vi "go to abort.vi"(0 "system status in":T2={"system state"=enum."Empty & Closed", "fuel level"=0.0, "LOX level"=0.0, "system warnings"={"oxidizer overpress"=FALSE, "oxidizer leak"=FALSE, "fuel overpress"=FALSE, "fuel leak"=FALSE}, "valves"={"fuel load"=FALSE, "fuel return"=FALSE, "fuel comb"=FALSE, "fuel dump"=FALSE, "LOX load"=FALSE, "LOX return"=FALSE, "LOX comb"=FALSE, "LOX dump"=FALSE}, "ignition"=FALSE}, 11 "rocket controls":T1, 13 "LOX over":bool, 15 "fuel over":bool) -> (4 "system status out":T2={"system state"=enum."Empty & Closed", "fuel level"=0.0, "LOX level"=0.0, "system warnings"={"oxidizer overpress"=FALSE, "oxidizer leak"=FALSE, "fuel overpress"=FALSE, "fuel leak"=FALSE}, "valves"={"fuel load"=FALSE, "fuel return"=FALSE, "fuel comb"=FALSE, "fuel dump"=FALSE, "LOX load"=FALSE, "LOX return"=FALSE, "LOX comb"=FALSE, "LOX dump"=FALSE}, "ignition"=FALSE})   [LabVIEW 2017]
doc: "This subVI handles the logic going to the abort state for the rocket engine simulation.\nIt sets the state enum to the abort state when the abort button is pushed, or if either overpressure sensor is set.\n\nPaul K Dixon\nP350\nCSUSB"
uses:
  typedefs/sysyem status.ctl
  typedefs/system state.ctl
  typedefs/rocket system warnings.ctl
  typedefs/user controls.ctl
panel:
  # "Standard\nProcedures"
  # "Alternate\nProcedures"
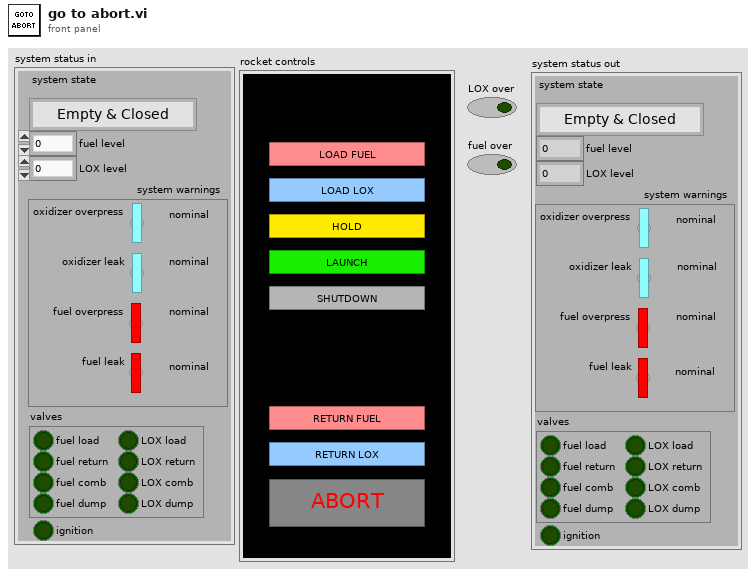
[diagram p1: front panel]
types:
  T1 = typedef "user controls.ctl" = cluster{"load fuel":bool, "load lox":bool, "hold":bool, "launch":bool, "shutdown":bool, "return fuel":bool, "return lox":bool, "abort":bool}
  T2 = typedef "sysyem status.ctl" = cluster{"system state":T3, "fuel level":dbl, "LOX level":dbl, "system warnings":T4, "valves":cluster{"fuel load":bool, "fuel return":bool, "fuel comb":bool, "fuel dump":bool, "LOX load":bool, "LOX return":bool, "LOX comb":bool, "LOX dump":bool}, "ignition":bool}
  T3 = typedef "system state.ctl" = enum16{"Hold", "Empty & Closed", "Launch", "Return Fuel", "Return LOX", "Loading Lox", "Loading Fuel", "Shutdown", "Abort"}
  T4 = typedef "rocket system warnings.ctl" = cluster{"oxidizer overpress":bool, "oxidizer leak":bool, "fuel overpress":bool, "fuel leak":bool}
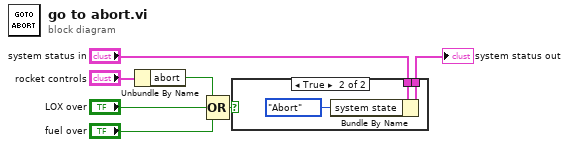
[diagram p0: block diagram]
diagram:
  n1 = Unbundle By Name("rocket controls") -> ("abort"=w1:bool)
  n2 = Compound Arithmetic op=OR(w1, "LOX over", "fuel over") -> (w5:bool)
  n3 = case shown="True" w5 {
    tunnel: "system status in" -> [w8 w11]
    tunnel: [w8 w10] -> w6
    frame False {
    }
    frame True {
      n4 = Bundle By Name(cluster=w11, "system state"=system_state."Abort") -> (w10:T2)
    }
  }
  "system status out" <- w6
